vi "Point getDistanceToLine.vi"(1 "point1":T1 {"y" format="%.2f"; "x" format="%.2f"}, 2 "line":T1[](array[typedef]) {"y" format="%.2f"; "x" format="%.2f"}, 5 "error in (no error)":errorcluster) -> (15 "minDistance":dbl format="%.2f", 19 "error out":errorcluster)   [LabVIEW 2014]
doc: "Gets the minimum distance to a line"
uses:
  <resource>/Framework/Providers/Open_GDS/UML/General/Point/Point Point2D.ctl
panel:
  # "size>=2"
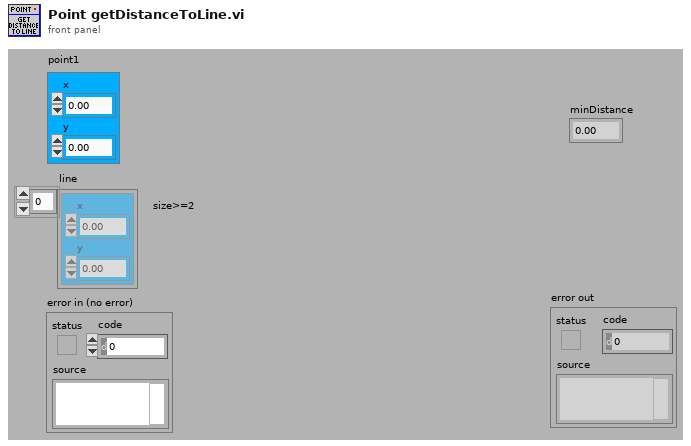
[diagram p1: front panel]
types:
  T1 = typedef "Point Point2D.ctl" = cluster{"x":dbl, "y":dbl}
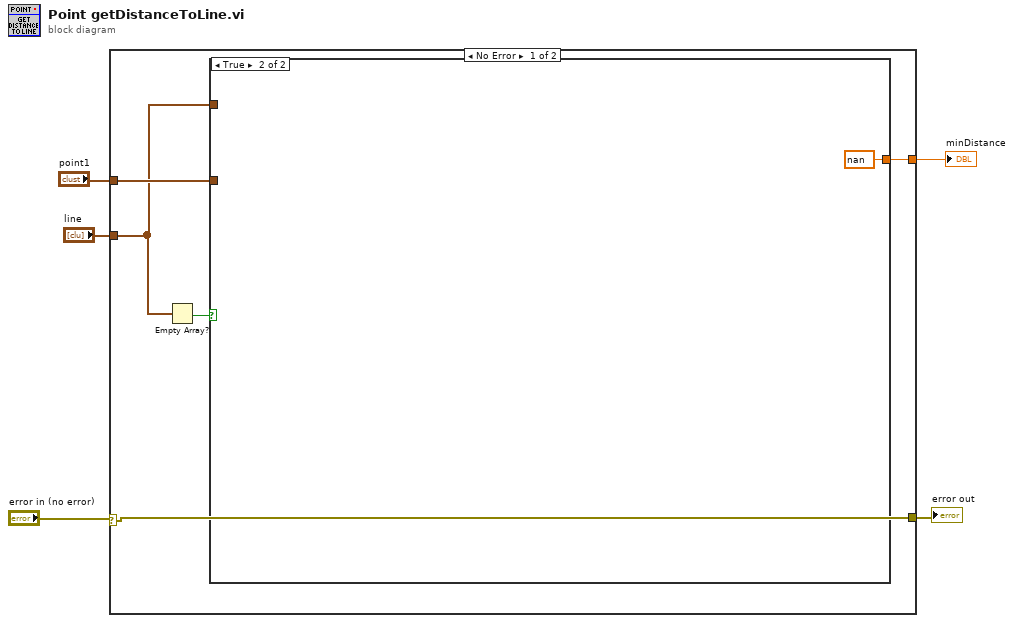
[diagram p0: block diagram]
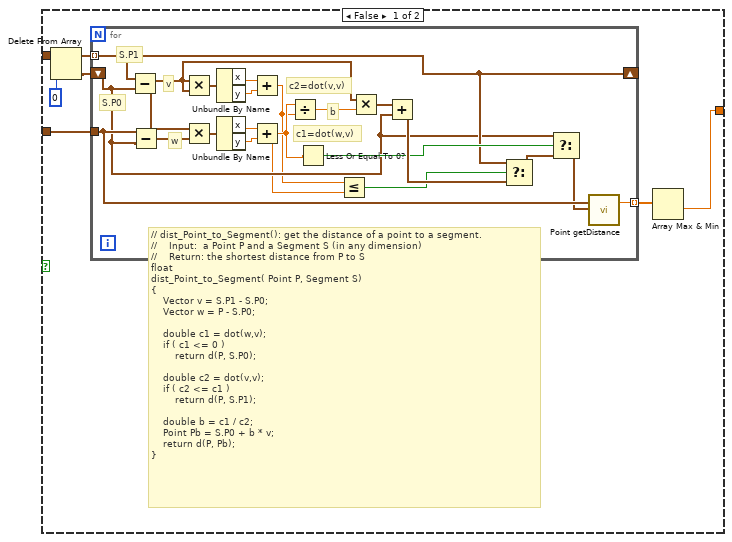
[diagram p2: hidden frame]
diagram:
  n1 = case shown="No Error" "error in (no error)" {
    selector: "error in (no error)" -> [w10 w40]
    tunnel: [w10 w40] -> w5
    tunnel: "point1" -> [w9 _]
    tunnel: "line" -> [w7 _]
    tunnel: [w8 _] -> w1
    frame No Error {
      n2 = Empty Array?(array=w7) -> (empty?=w6:bool)
      n3 = case shown="True" w6 {
        tunnel: w9 -> [w14 _]
        tunnel: [w12 nan] -> w8
        tunnel: w7 -> [w11 _]
        frame False {
          # "// dist_Point_to_Segment(): get the distance of a point to a segment.\n//    Input:  a Point P and a Segment S (in any dimension)\n//    Return: the shortest distance from P to S\nfloat\ndist_Point_to_Segment( Point P, Segment S)\n{\n    Vector v = S.P1 - S.P0;\n    Vector w = P - S.P0;\n\n    double c1 = dot(w,v);\n    if ( c1 <= 0 )\n        return d(P, S.P0);\n\n    double c2 = dot(v,v);\n    if ( c2 <= c1 )\n        return d(P, S.P1);\n\n    double b = c1 / c2;\n    Point Pb = S.P0 + b * v;\n    return d(P, Pb);\n}"
          n4 = Delete From Array(array=w11, index=0) -> (deleted portion=w15:T1, array with subset deleted=w16:T1[])  [unwired: 1 in]
          n5 = for {
            tunnel: w16 -> [w22] mode=indexing
            shift-right: [w22] -> _
            shift-left: w15 -> [w21]
            tunnel: w14 -> [w28]
            tunnel: [w27] -> w13 mode=indexing
            # "S.P1"
            # "S.P0"
            # "b"
            # "c2=dot(v,v)"
            # "c1=dot(w,v)"
            # "w"
            # "v"
            n6 = Subtract(x=w22, y=w21) -> (x-y=w30:T1)
            n7 = Subtract(x=w28, y=w21) -> (x-y=w38:T1)
            n8 = Multiply(x=w30, y=w30) -> (x*y=w32:T1)
            n9 = Multiply(x=w30, y=w38) -> (x*y=w37:T1)
            n10 = Unbundle By Name(w32) -> ("x"=w34:dbl, "y"=w33:dbl)
            n11 = Unbundle By Name(w37) -> ("x"=w35:dbl, "y"=w36:dbl)
            n12 = Add(x=w34, y=w33) -> (x+y=w18:dbl)
            n13 = Add(x=w35, y=w36) -> (x+y=w19:dbl)
            n14 = Divide(x=w19, y=w18) -> (x/y=w31:dbl)
            n15 = Less Or Equal To 0?(x=w19) -> (x <= 0?=w23:bool)
            n16 = Less Or Equal?(x=w18, y=w19) -> (x <= y?=w20:bool)
            n17 = Multiply(x=w30, y=w31) -> (x*y=w29:T1)
            n18 = Add(x=w29, y=w21) -> (x+y=w24:T1)
            n19 = Select(t=w22, s=w20, f=w24) -> (s? t:f=w25:T1)
            n20 = Select(t=w21, s=w23, f=w25) -> (s? t:f=w26:T1)
            n21 = call <resource>:"Point getDistance.vi"("point1"=w28, "point2"=w26) -> ("distance"=w27:dbl)  [unwired: 1 in, 16 out]
          }
          n22 = Array Max & Min(array=w13) -> (min value=w12:dbl)  [unwired: 3 out]
        }
        frame True {
        }
      }
    }
    frame Error {
    }
  }
  "error out" <- w5
  "minDistance" <- w1
